vi "fbk_timeout_error.vi"(4 "INIT mode":enum16{"online", "demo", "compile"}(ring), 6 "INIT? (F)":bool, 7 "timeout?":bool, 8 "error in (no error)":errorcluster, 9 "argument":string, 10 "channel":string, 11 "timeout time":dbl format="%#_13g") -> (0 "error out":errorcluster)   [LabVIEW 2017]
uses:
  error_codes_labview_colossus.ctl
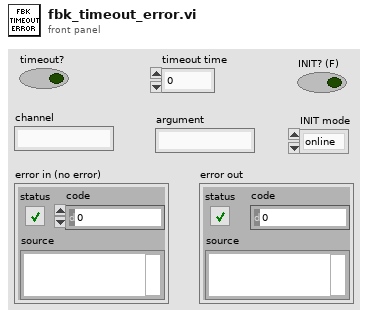
[diagram p1: front panel]
types:
  T1 = typedef "error_codes_labview_colossus.ctl" = i32
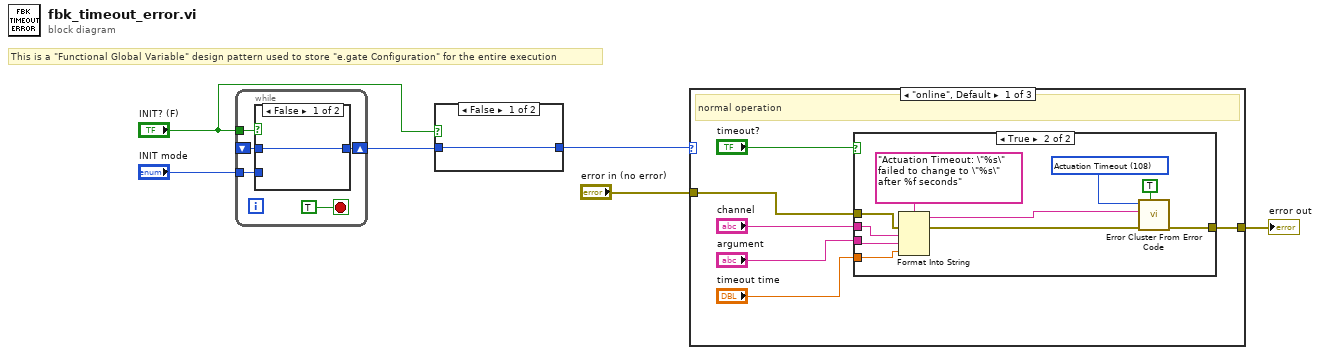
[diagram p0: block diagram]
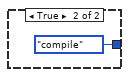
[diagram p2: hidden frame]
diagram:
  # "This is a \"Functional Global Variable\" design pattern used to store \"e.gate Configuration\" for the entire execution"
  n1 = while {
    tunnel: "INIT? (F)" -> [w10]
    shift-right: [w9] -> w3
    shift-left: _ -> [w8]
    tunnel: "INIT mode" -> [w7]
    stop <- TRUE stop-if-true
    n2 = case shown="False" w10 {
      tunnel: [w12 w13] -> w9
      tunnel: w8 -> [w12 _]
      tunnel: w7 -> [_ w13]
      frame False {
      }
      frame True {
      }
    }
  }
  n3 = case shown="False" "INIT? (F)" {
    tunnel: w3 -> [w14 _]
    tunnel: [w14 enum16{"online", "demo", "compile"}."compile" ("INIT mode")] -> w2
    frame False {
    }
    frame True {
    }
  }
  n4 = case shown="\"online\", Default" w2 {
    tunnel: [w18 w33 w34] -> w6
    tunnel: "error in (no error)" -> [w17 w33 w34]
    frame "online", Default {
      # "normal operation"
      n5 = case shown="True" "timeout?" {
        tunnel: w17 -> [w22 w27]
        tunnel: [w22 w26] -> w18
        tunnel: "channel" -> [_ w25]
        tunnel: "argument" -> [_ w24]
        tunnel: "timeout time" -> [_ w23]
        frame False {
        }
        frame True {
          w31 = T1 108 items=["No error", "Argument error", "Memory is full", "Out of zone", "End of file", "File already open", "Generic file I/O error", "File not found", "File permission error", "Disk is full", "Duplicate path", "Too many files open", "System feature not enabled", "Resource file not found", "Cannot add resource", "Resource not found", "Image not found", "Image memory error", "Pen does not exist", "Config type invalid", "Config token not found", "Config parse error", "Config memory error", "Bad external code format", "Bad external code offset", "External code not present", "Null window", "Destroy window error", "Null menu", "Print aborted", "Bad print record", "Print driver error", "Windows error during printing", "Memory error during printing", "Print dialog error", "Generic print error", "Invalid device refnum", "Device not found", "Device parameter error", "Device unit error", "Cannot open device", "Device call aborted", "Generic error", "Cancelled by user", "Object ID too low", "Object ID too high", "Object not in heap", "Unknown heap", "Unknown object (invalid DefProc)", "Unknown object (DefProc not in table)", "Message out of range", "Invalid (null) method", "Unknown message", "Manager call not supported", "Bad address", "Network operation in progress", "Network operation timed out", "Connection is busy", "Network attribute not supported", "Network error", "Address in use", "System out of memory", "Connection aborted", "Connection refused", "Not connected", "Already connected", "Connection closed", "Initialization error (interapplication manager)", "Bad occurrence", "Wait on unbound occurrence handler", "Occurrence queue overflow", "Datalog type conflict", "Unused", "Unrecognized type (interapplication manager)", "Memory corrupt", "Failed to make temporary DLL", "Old CIN version", "Drag socket not found", "Failed to load drop-object", "Failed to register OLE object", "Failed to release OLE object", "Format specifier type mismatch", "Unknown format specifier", "Too few format specifiers", "Too many format specifiers", "Scan failed", "Newer CIN version", "Error converting to variant", "Runtime menu error", "Password tampered", "Variant attribute not found", "Incompatible variant data type", "Event data is not available", "Event Store is not present", "Occurrence is not found", "Event Queue is not created", "Event info is not available", "Refnum passed is NULL", "Error retrieving Class GUID", "Error retrieving CoClass GUID", "Error retrieving TypeLib GUID.", "Bad built application magic bytes.", "Specific driver is different from the specific driver associated with the Logical Name.", "There is no session opened to the class driver.", "Max Error", "MAX - Error with config objects", "MAX - Error loading configuration", "MAX - Group not supported", "Actuation Timeout", "Invalid Argument", "Invalid Config Key"]
          n6 = Format Into String(format string="Actuation Timeout: \"%s\" failed to change to \"%s\" after %f seconds" ("message"), error in=w27, w25, w24, w23) -> (resulting string=w30:string, error out=w29:errorcluster)  [unwired: 1 in]
          n7 = call <vilib>:"Error Cluster From Error Code.vi"("show call chain? (False)"=TRUE, "error in (no error)"=w29, "error message (\"\")"=w30, "error code (0)"=w31) -> ("error out"=w26:errorcluster)  [unwired: 5 in]
        }
      }
    }
    frame "demo" {
      # "demo mode"
    }
    frame "compile" {
      # "compile mode"
    }
  }
  "error out" <- w6
